vi "durationOscillation.vi"(1 "valesAmplitude2":dbl, 2 "timeValesLocation1":dbl, 3 "valesAmplitude1":dbl, 4 "timeValesLocation2":dbl) -> (0 "durationOscilation":dbl)   [LabVIEW 2012]
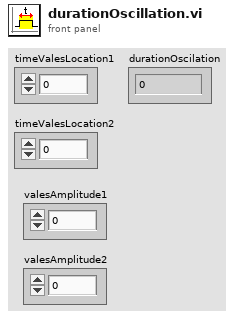
[diagram p1: front panel]
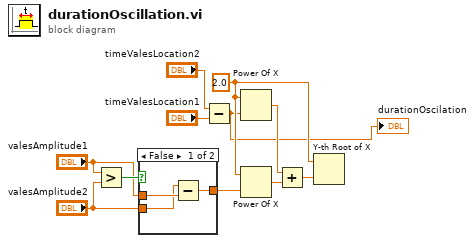
[diagram p0: block diagram]
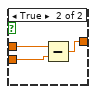
[diagram p2: hidden frame]
diagram:
  w11 = 2.0 ("y")
  n1 = Greater?(x="valesAmplitude1", y="valesAmplitude2") -> (0:w5:bool)
  n2 = case shown="False" w5 {
    tunnel: "valesAmplitude1" -> [w14 w17]
    tunnel: "valesAmplitude2" -> [w13 w16]
    tunnel: [w12 w15] -> w4
    frame False {
      n3 = Subtract(x=w13, y=w14) -> (x-y=w12:dbl)
    }
    frame True {
      n4 = Subtract(x=w17, y=w16) -> (x-y=w15:dbl)
    }
  }
  n5 = Subtract(x="timeValesLocation2", y="timeValesLocation1") -> (x-y=w1:dbl)
  "durationOscilation" <- w1
  n6 = Power Of X(1:w1, 2:w11) -> (0:w8:dbl)
  n7 = Power Of X(1:w4, 2:w11) -> (0:w9:dbl)
  n8 = Add(x=w8, y=w9) -> (x+y=w10:dbl)
  n9 = Y-th Root of X(1:w10, 2:w11) -> ()  [unwired: 1 out]
